vi "osa_parse test and reset result.vi"(8 "error in (no error)":errorcluster, 11 "serial response in":string) -> (0 "error out":errorcluster, 3 "test/reset result":bool)   [LabVIEW 2021]
uses:
  <vilib>/ErrorRing/Error Ring.xnode
panel:
  # "OSA subVI: parse test/reset result, return boolean array"
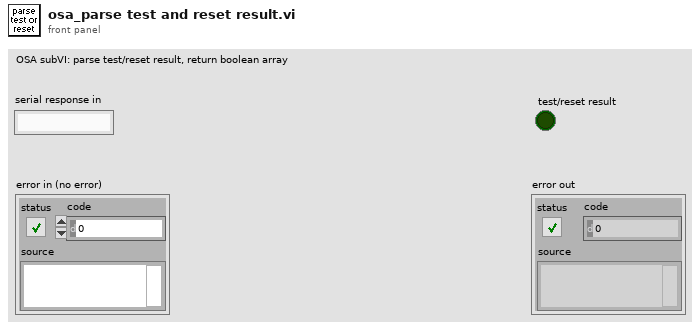
[diagram p1: front panel]
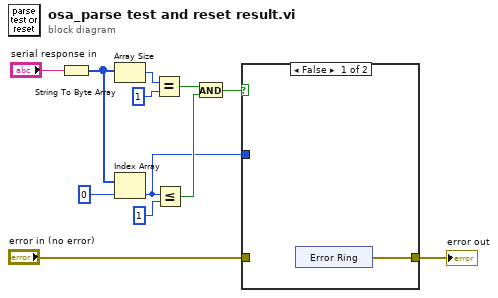
[diagram p0: block diagram]
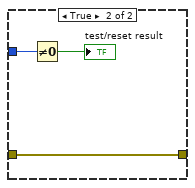
[diagram p2: hidden frame]
diagram:
  n1 = String To Byte Array(string="serial response in") -> (unsigned byte array=w10:u8[])
  n2 = Array Size(array=w10) -> (size(s)=w11:i32)
  n3 = Index Array(array=w10, index=0) -> (element=w3:u8)
  n4 = Equal?(x=w11, y=1) -> (x = y?=w5:bool)
  n5 = Less Or Equal?(x=w3, y=u8 1) -> (x <= y?=w6:bool)
  n6 = And(x=w5, y=w6) -> (x .and. y?=w4:bool)
  n7 = case shown="False" w4 {
    tunnel: w3 -> [_ w17]
    tunnel: "error in (no error)" -> [_ w15]
    tunnel: [w13 w15] -> w1
    frame False {
      n8 = xnode "Error Ring"() -> ("error out"=w13:errorcluster)
    }
    frame True {
      n9 = Not Equal To 0?(x=w17) -> (x != 0?=→"test/reset result":bool)
    }
  }
  "error out" <- w1
